vi "Split Extension.vi"(11 "Filename":string) -> (2 "Extension":string, 3 "Name":string)   [LabVIEW 2011]
doc: "Takes a filename and returns the name and extension.\n\n\nVersion 1.0 - 10/20/2009\n\nPhaeron, Inc.\nwww.phaeron.com\ninfo@phaeron.com"
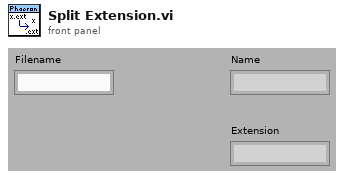
[diagram p1: front panel]
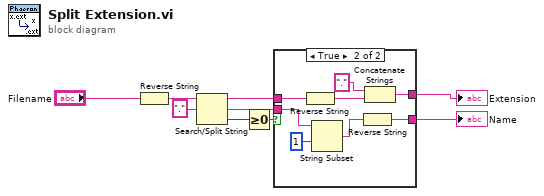
[diagram p0: block diagram]
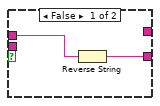
[diagram p2: hidden frame]
diagram:
  n1 = Reverse String(1:"Filename") -> (0:w5:string)
  n2 = Search/Split String(string=w5, search string/char (-)="." ("string")) -> (substring before match=w4:string, match + rest of string=w3:string, offset of match=w2:i32)  [unwired: 1 in]
  n3 = Greater Or Equal To 0?(x=w2) -> (x >= 0?=w1:bool)
  n4 = case shown="True" w1 {
    tunnel: w4 -> [w11 w18]
    tunnel: [_ w17] -> w8
    tunnel: w3 -> [_ w14]
    tunnel: [w10 w12] -> w7
    frame False {
      n5 = Reverse String(1:w11) -> (0:w10:string)
    }
    frame True {
      n6 = Reverse String(1:w18) -> (0:w19:string)
      n7 = String Subset(string=w14, offset (0)=1) -> (substring=w13:string)  [unwired: 1 in]
      n8 = Reverse String(1:w13) -> (0:w12:string)
      n9 = Concatenate Strings("." ("string"), w19) -> (w17:string)
    }
  }
  "Name" <- w7
  "Extension" <- w8
